vi "ExecuteButtonAction.vi"(8 "ErrorIn":errorcluster, 9 "WaitForReply":bool, 10 "Command":string, 11 "ReferenceIn":refnum<class "VerticalButtonBar.lvclass">) -> (0 "ErrorOut":errorcluster, 3 "ReferenceIn":refnum<class "VerticalButtonBar.lvclass">)   [LabVIEW 2021, in "VerticalButtonBar.lvclass"]
uses:
  VerticalButtonBar.lvclass
  VerticalButtonBar.lvclass/VerticalButtonBar.ctl
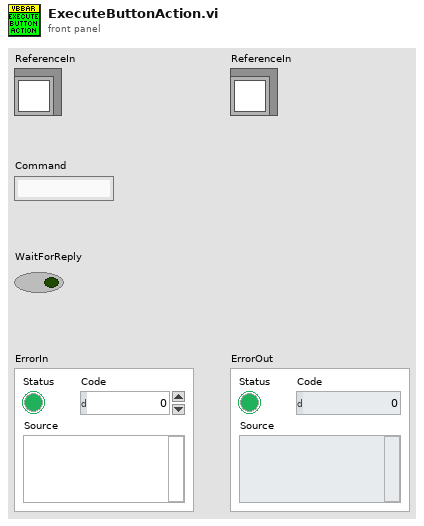
[diagram p1: front panel]
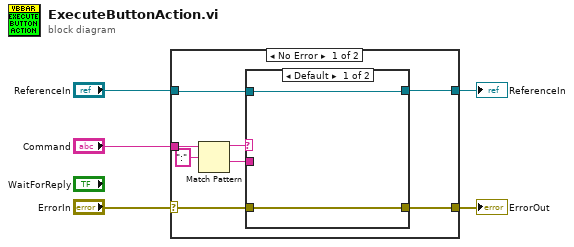
[diagram p0: block diagram]
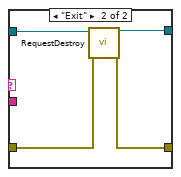
[diagram p2: hidden frame]
diagram:
  n1 = case shown="No Error" "ErrorIn" {
    selector: "ErrorIn" -> [w13 w21]
    tunnel: [w12 w21] -> w4
    tunnel: [w10 w20] -> w2
    tunnel: "ReferenceIn" -> [w11 w20]
    tunnel: "Command" -> [w9 _]
    frame No Error {
      n2 = Match Pattern(string=w9, regular expression=":") -> (before substring=w8:string, after substring=w6:string)  [unwired: 1 in, 2 out]
      n3 = case shown="Default" w8 {
        tunnel: w11 -> [w14 w17]
        tunnel: [w14 w16] -> w10
        tunnel: w6 -> [_ _]
        tunnel: [w15 w18] -> w12
        tunnel: w13 -> [w15 w19]
        frame Default {
        }
        frame "Exit" {
          n4 = call "RequestDestroy.vi"("ErrorIn"=w19, "ReferenceIn"=w17) -> ("ErrorOut"=w18:errorcluster, "ReferenceOut"=w16:refnum<class "VerticalButtonBar.lvclass">)  [unwired: 8 in]
        }
      }
    }
    frame Error {
    }
  }
  "ErrorOut" <- w4
  "ReferenceIn" <- w2
